vi "Write Coils.vi"(6 "timeout ms (1000)":i32=1000, 8 "error in (no error)":errorcluster, 9 "Value":bool[](array[boolean]), 10 "Start Address":u16, 11 "TCP Network Connection in":refnum<k5>) -> (0 "error out":errorcluster, 3 "TCP Network Connection out":refnum<k5>)   [LabVIEW 2023, in "Modbus TCP Micro.lvlib"]
uses:
  Modbus TCP Micro.lvlib
  Modbus Functions.ctl
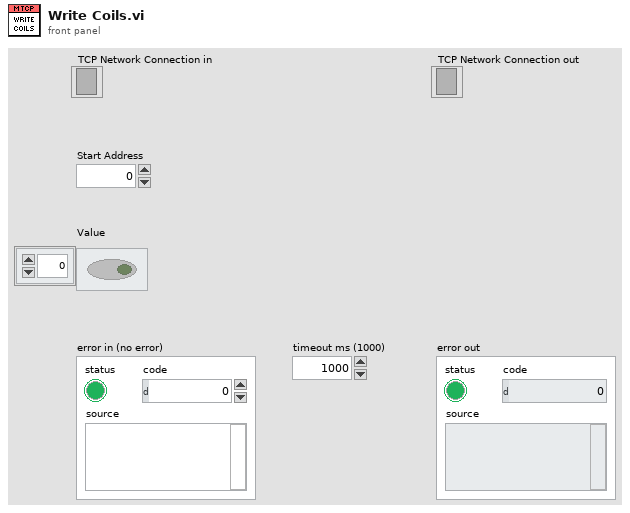
[diagram p1: front panel]
types:
  T1 = typedef "Modbus TCP Micro.lvlib/Modbus Functions.ctl" = u8
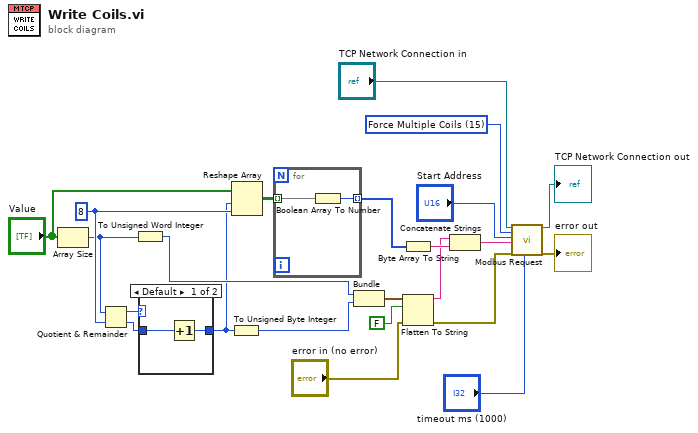
[diagram p0: block diagram]
diagram:
  w3 = T1 15 items=["None"=0, "Read Coil Status"=1, "Read Input Status"=2, "Read Holding Registers"=3, "Read Input Registers"=4, "Force Single Coil"=5, "Preset Single Register"=6, "Force Multiple Coils"=15, "Preset Multiple Registers"=16] ("Function Codes")
  w17 = 8 ("y")
  n1 = Array Size(array="Value") -> (size(s)=w14:i32)
  n2 = Quotient & Remainder(x=w14, y=w17) -> (x-y*floor(x/y)=w20:i32, floor(x/y)=w19:i32)
  n3 = To Unsigned Word Integer(number=w14) -> (unsigned 16bit integer=w13:u16)
  n4 = case shown="Default" w20 {
    tunnel: w19 -> [w25 w26]
    tunnel: [w24 w26] -> w11
    frame Default {
      n5 = Increment(x=w25) -> (x+1=w24:i32)
    }
    frame 0 {
    }
  }
  n6 = To Unsigned Byte Integer(number=w11) -> (unsigned 8bit integer=w10:u8)
  n7 = Reshape Array("Value", w11, w17) -> (w16:bool[][])
  n8 = for {
    tunnel: w16 -> [w28] mode=indexing
    tunnel: [w27] -> w12 mode=indexing
    n9 = Boolean Array To Number(Boolean array=w28) -> (number=w27:u8)
  }
  n10 = Bundle(w13, w10) -> (w9:cluster{u16, u8})  [unwired: 1 in]
  n11 = Byte Array To String(unsigned byte array=w12) -> (string=w15:string)
  n12 = Flatten To String(anything=w9, prepend array or string size? (T)=FALSE, error in (no error)="error in (no error)") -> (data string=w4:string, error out=w7:errorcluster)  [unwired: 1 in, 1 out]
  n13 = Concatenate Strings(w4, w15) -> (w5:string)
  n14 = call "Modbus Request.vi"("TCP Network Connection in"="TCP Network Connection in", "Function Codes"=w3, "Start Address"="Start Address", "Payload"=w5, "error in (no error)"=w7, "timeout ms (1000)"="timeout ms (1000)") -> ("TCP Network Connection out"=→"TCP Network Connection out":refnum<k5>, "error out"=→"error out":errorcluster)  [unwired: 8 in, 4 out]
